vi "simx Load UI.vi"(0 "clientID":i32, 1 "uiHandles":i32, 5 "uiPathAndName":string, 7 "options":u8, 9 "count":i32, 11 "error in (no error)":errorcluster, 12 "operationMode":i32) -> (3 "uiHandles out":i32, 4 "function return":i32, 10 "count out":i32, 15 "error out":errorcluster)   [LabVIEW 2019, in "PXL_V-REP.lvlib"]
doc: "EXTAPI_DLLEXPORT simxInt simxLoadUI(simxInt clientID,const simxChar* uiPathAndName,simxUChar options,simxInt* count,simxInt** uiHandles,simxInt operationMode);"
uses:
  PXL_V-REP.lvlib
  <userlib>/V-REP/remoteApi.dll
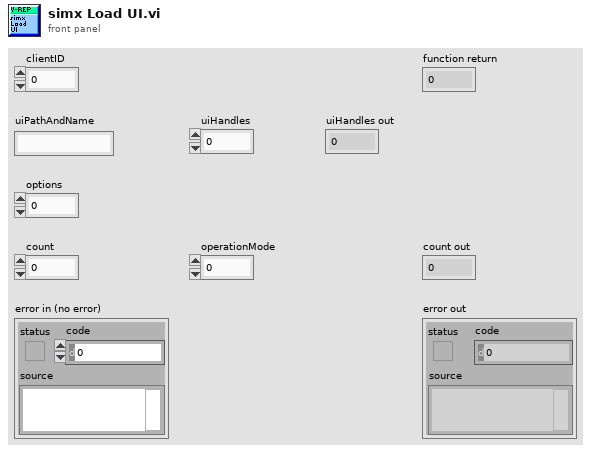
[diagram p1: front panel]
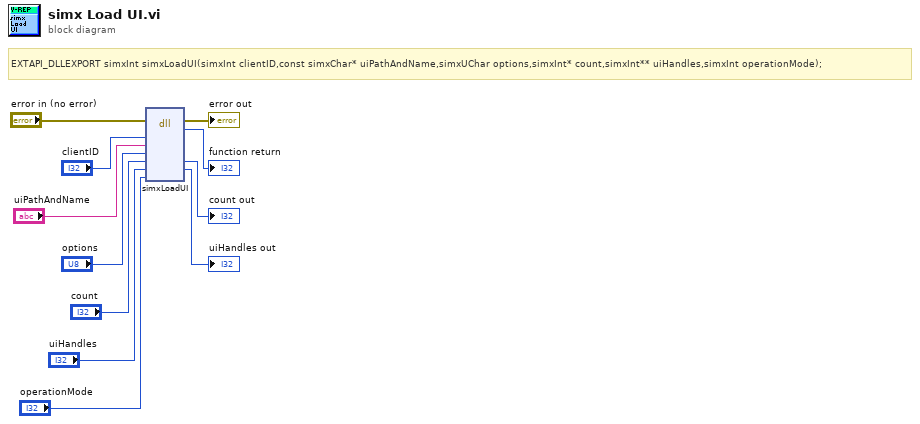
[diagram p0: block diagram]
diagram:
  # "EXTAPI_DLLEXPORT simxInt simxLoadUI(simxInt clientID,const simxChar* uiPathAndName,simxUChar options,simxInt* count,simxInt** uiHandles,simxInt operationMode);"
  n1 = dll-call lib="C:/Program Files (x86)/National Instruments/LabVIEW 2019/user.lib/V-REP/remoteApi.*" fn="simxLoadUI"(error in="error in (no error)", "clientID"="clientID", "uiPathAndName"="uiPathAndName", "options"="options", "count"="count", "uiHandles"="uiHandles", "operationMode"="operationMode") -> (error out=→"error out":errorcluster, →"function return":i32, "count"=→"count out":i32, "uiHandles"=→"uiHandles out":i32)  [unwired: 6 in, 1 out]
